vi "Set PID Gains.vi"(8 "error in (no error)":errorcluster, 10 "PID gains":T1, 11 "PID Loop in":refnum<class "PID Loop.lvclass">) -> (0 "error out":errorcluster, 3 "PID Loop out":refnum<class "PID Loop.lvclass">)   [LabVIEW 2024, in "PID Loop.lvlib" / "PID Loop.lvclass"]
uses:
  PID Loop.lvclass
  PID Loop.lvclass/PID Loop.ctl
  PID/PID/PID.lvclass
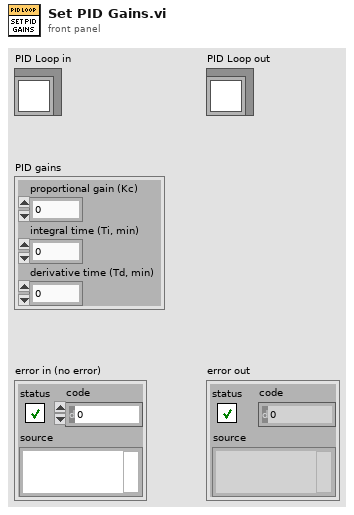
[diagram p1: front panel]
types:
  T1 = cluster{"proportional gain (Kc)":dbl, "integral time (Ti, min)":dbl, "derivative time (Td, min)":dbl}
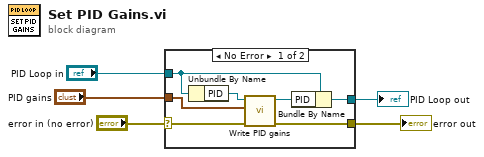
[diagram p0: block diagram]
diagram:
  n1 = case shown="No Error" "error in (no error)" {
    selector: "error in (no error)" -> [w7 w14]
    tunnel: [w6 w14] -> w4
    tunnel: [w11 w13] -> w2
    tunnel: "PID Loop in" -> [w12 w13]
    tunnel: "PID gains" -> [w8 _]
    frame No Error {
      n2 = Unbundle By Name(w12) -> ("PID"=w10:refnum<class "PID.lvclass">)
      n3 = call-dynamic "Write PID gains.vi"("error in (no error)"=w7, "PID gains"=w8, "PID in"=w10) -> ("error out"=w6:errorcluster, "PID out"=w9:refnum<class "PID.lvclass">)  [unwired: 7 in]
      n4 = Bundle By Name(cluster=w12, "PID"=w9) -> (w11:refnum<class "PID Loop.lvclass">)
    }
    frame Error {
    }
  }
  "error out" <- w4
  "PID Loop out" <- w2
